vi "DSF.Engine.Interface.RT FIFO.Delete.16B.vi"(8 "error in (no error)":errorcluster, 11 "RT FIFO":T1) -> (0 "error out":errorcluster)   [LabVIEW 2017, in "DSF.Engine.lvlib" / "DSF.Engine.Interface.lvclass"]
uses:
  DSF.Engine.Interface.lvclass
  DSF.Engine.Interface.RT FIFO.Ref.16B.ctl
  DSF.Engine.Interface.RT FIFO.Data.16B.ctl
  DSF.Engine.Interface.RT FIFO.Payload.16B.ctl
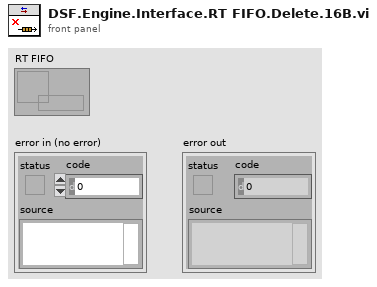
[diagram p1: front panel]
types:
  T1 = typedef "DSF.Engine.lvlib/DSF.Engine.Interface.lvclass/DSF.Engine.Interface.RT FIFO.Ref.16B.ctl" = refnum<k33>
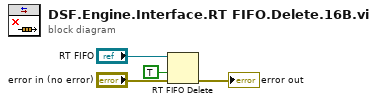
[diagram p0: block diagram]
diagram:
  n1 = RT FIFO Delete(0:"RT FIFO", 2:TRUE ("force destroy? (F)"), 3:"error in (no error)") -> (11:→"error out":errorcluster)
